vi "All Reservations.vi"(2 "Reset":bool, 3 "Line to add":string) -> (0 "Line added?":bool, 1 "Lines reserved":string[](array[string]))   [LabVIEW 2015]
doc: "Keeps track of which lines or other resources have been reserved. Uses strings so that resources of different types (e.g. hardware lines and also logfiles) can be both be kept track of.\n\nSome use cases:\nReset list: wire TRUE to [Reset]\nSee list: no inputs, read [Lines reserved] output\nReserve new line: wire [Line to add] input, check [Line added?] output to see if it was able to be reserved.\n\nIf you want to reserve multiple hardware lines, make sure you do them one-by-one, otherwise the collision checking won't work!"
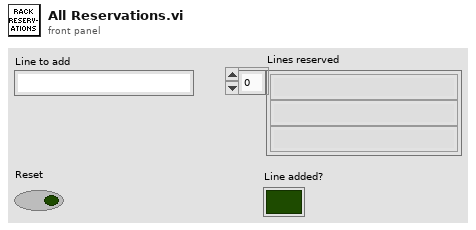
[diagram p1: front panel]
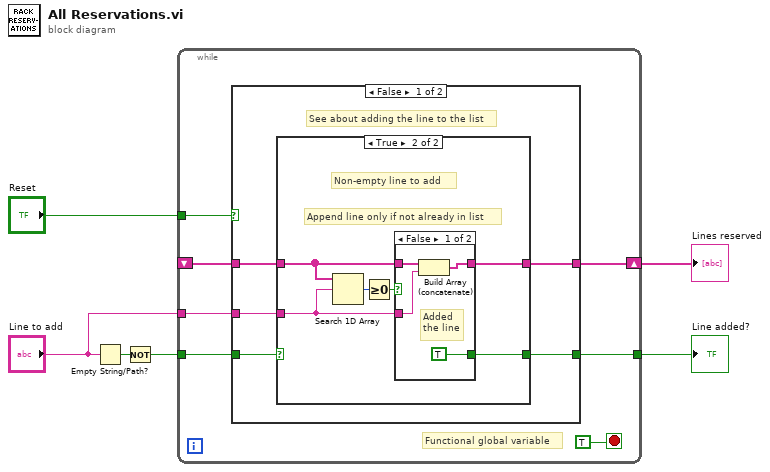
[diagram p0: block diagram]
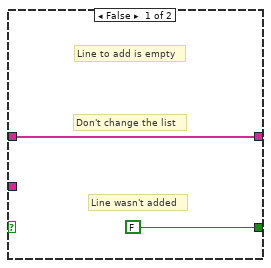
[diagram p2: hidden frame]
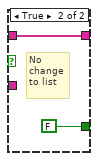
[diagram p3: hidden frame]
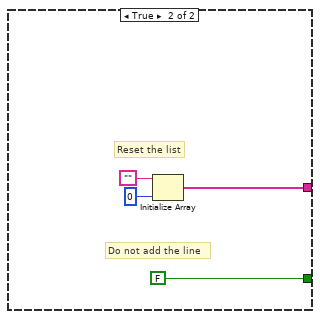
[diagram p4: hidden frame]
diagram:
  n1 = Empty String/Path?(string/path="Line to add") -> (empty?=w6:bool)
  n2 = Not(x=w6) -> (.not. x?=w5:bool)
  n3 = while {
    tunnel: w5 -> [w13]
    tunnel: [w12] -> w4
    tunnel: "Reset" -> [w11]
    shift-right: [w10] -> w2
    shift-left: _ -> [w8]
    tunnel: "Line to add" -> [w7]
    stop <- TRUE ("stop") stop-if-true
    # "Functional global variable"
    n4 = case shown="False" w11 {
      tunnel: w13 -> [w18 _]
      tunnel: [w17 FALSE] -> w12
      tunnel: [w16 w34] -> w10
      tunnel: w8 -> [w15 _]
      tunnel: w7 -> [w14 _]
      frame False {
        # "See about adding the line to the list"
        n5 = case shown="True" w18 {
          tunnel: [FALSE w21] -> w17
          tunnel: [w20 w23] -> w16
          tunnel: w15 -> [w20 w24]
          tunnel: w14 -> [_ w22]
          frame False {
            # "Line wasn't added"
            # "Don't change the list"
            # "Line to add is empty"
          }
          frame True {
            # "Append line only if not already in list"
            # "Non-empty line to add"
            n6 = Search 1D Array(1D array=w24, element=w22) -> (index of element=w26:i32)  [unwired: 1 in]
            n7 = Greater Or Equal To 0?(x=w26) -> (x >= 0?=w25:bool)
            n8 = case shown="False" w25 {
              tunnel: w24 -> [w30 w32]
              tunnel: [w29 w32] -> w23
              tunnel: w22 -> [w28 _]
              tunnel: [TRUE FALSE] -> w21
              frame False {
                # "Added\nthe line"
                n9 = Build Array (concatenate)(w30, w28) -> (w29:string[])
              }
              frame True {
                # "No\nchange\nto list"
              }
            }
          }
        }
      }
      frame True {
        # "Do not add the line"
        # "Reset the list"
        n10 = Initialize Array("", 0 ("dimension size")) -> (w34:string[])
      }
    }
  }
  "Lines reserved" <- w2
  "Line added?" <- w4
